vi "getVSource.vi"(8 "error in (no error)":errorcluster, 11 "Electrometer in":refnum<class "Electrometer.lvclass">) -> (0 "error out":errorcluster, 2 "Voltaje":string, 3 "Electrometer out":refnum<class "Electrometer.lvclass">)   [LabVIEW 2016, in "Electrometer.lvclass"]
uses:
  Electrometer.lvclass
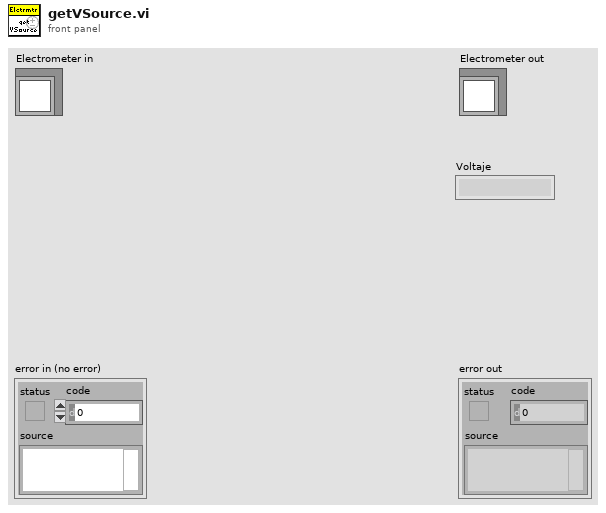
[diagram p1: front panel]
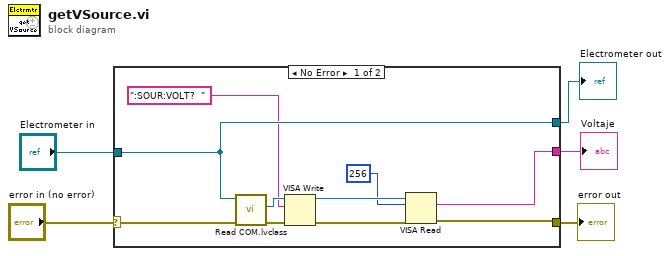
[diagram p0: block diagram]
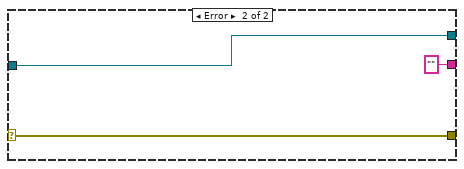
[diagram p2: hidden frame]
diagram:
  n1 = case shown="No Error" "error in (no error)" {
    selector: "error in (no error)" -> [w15 w18]
    tunnel: [w10 w18] -> w4
    tunnel: [w12 w17] -> w2
    tunnel: "Electrometer in" -> [w12 w17]
    tunnel: [w7 "" ("read buffer")] -> w1
    frame No Error {
      n2 = call "Read COM.lvclass.vi"("error in (no error)"=w15, "Electrometer in"=w12) -> ("error out"=w13:errorcluster, "VISA"=w14:refnum<visa-resource-name>)  [unwired: 7 in, 1 out]
      n3 = VISA Write(VISA resource name=w14, write buffer=":SOUR:VOLT?  " ("string"), error in (no error)=w13) -> (VISA resource name out=w9:refnum<visa-resource-name>, error out=w11:errorcluster)  [unwired: 1 out]
      n4 = VISA Read(VISA resource name=w9, byte count=u32 256, error in (no error)=w11) -> (read buffer=w7:string, error out=w10:errorcluster)  [unwired: 2 out]
    }
    frame Error {
    }
  }
  "error out" <- w4
  "Electrometer out" <- w2
  "Voltaje" <- w1
